vi "PCO_Live.vi"(7 "Message Data":variant, 8 "entrée d'erreur (pas d'erreur)":errorcluster, 9 "Display loop":refnum<queue>, 10 "dup Message Queue":refnum<queue>, 11 "Camera en entrée":refnum<class "Camera.lvclass">) -> (0 "sortie d'erreur":errorcluster, 3 "Camera en sortie":refnum<class "Camera.lvclass">)   [LabVIEW 2026]
uses:
  QMH/Message Queue/Message Cluster.ctl
  <instrlib>/PCO_SDK/File Group 0/vi.lib/Excelitas PCO GmbH/pco.labview/camera/Camera.lvclass
  <instrlib>/PCO_SDK/File Group 0/vi.lib/Excelitas PCO GmbH/pco.labview/camera/Controls/binning.ctl
  Controls/PCO_Config.ctl
  Controls/TypeDef_FGV.ctl
  QMH/Message Queue/Enqueue Message (Single).vi
  QMH/Message Queue/Message Queue.lvlib
panel:
  out "cluster de sortie":T2 {"binning"."mode" items=["sum", "average"]}
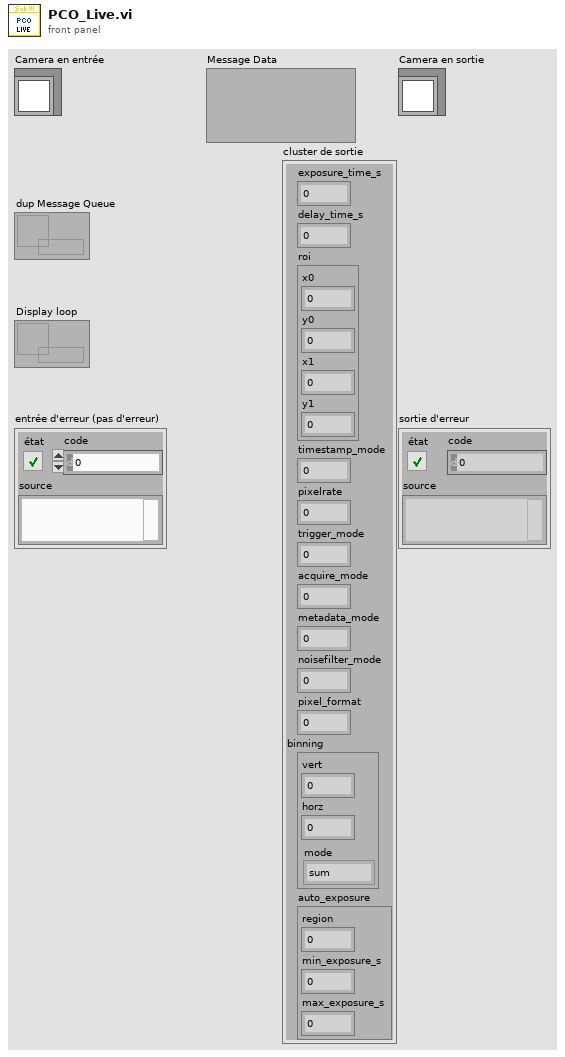
[diagram p1: front panel]
types:
  T1 = typedef "Camera.lvclass/binning.ctl" = cluster{"vert":u16, "horz":u16, "mode":u16}
  T2 = cluster{"exposure_time_s":dbl, "delay_time_s":dbl, "roi":cluster{"x0":u64, "y0":u64, "x1":u64, "y1":u64}, "timestamp_mode":u16, "pixelrate":u32, "trigger_mode":u16, "acquire_mode":u16, "metadata_mode":u16, "noisefilter_mode":u16, "pixel_format":u32, "binning":T1, "auto_exposure":cluster{"region":u16, "min_exposure_s":dbl, "max_exposure_s":dbl}}
  T3 = typedef "PCO_Config.ctl" = cluster{"Exposure time (s)":dbl, "TriggerMode":u16, "ROI X0":u16, "ROI Y0":u16, "ROI X1":u16, "ROI Y1":u16, "Binning":u8}
  T4 = enum16{"sequence", "sequence non blocking", "ring buffer", "fifo", "sequence_dpcore", "sequence_non_blocking_dpcore", "ring_buffer_dpcore", "fifo_dpcore", "tif", "multitif", "pcoraw", "b16", "dicom", "multidicom", "camram_ring", "camram_segment"}
  T5 = typedef "TypeDef_FGV.ctl" = enum16{"Initialize", "Write", "Read"}
  T6 = enum16{"Undefined", "Mono8", "Mono16", "BGRA8", "RGBA8", "BGRA16", "RGBA16", "CompressedMono8"}
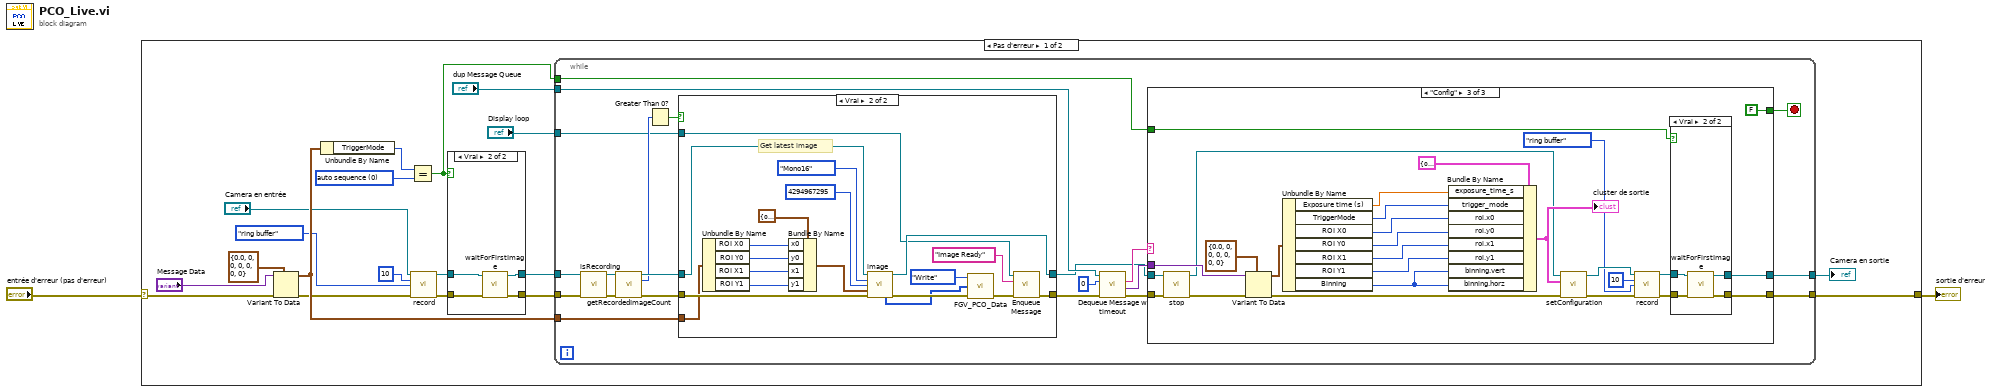
[diagram p0: block diagram]
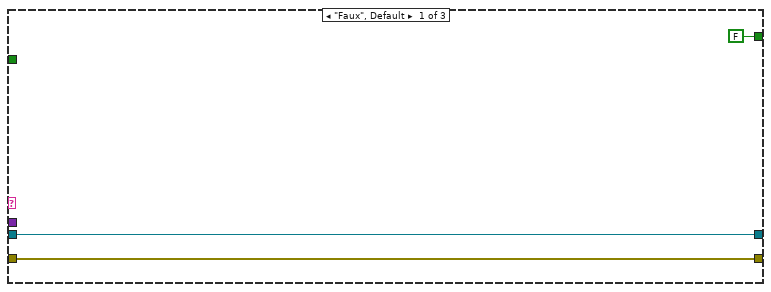
[diagram p2: hidden frame]
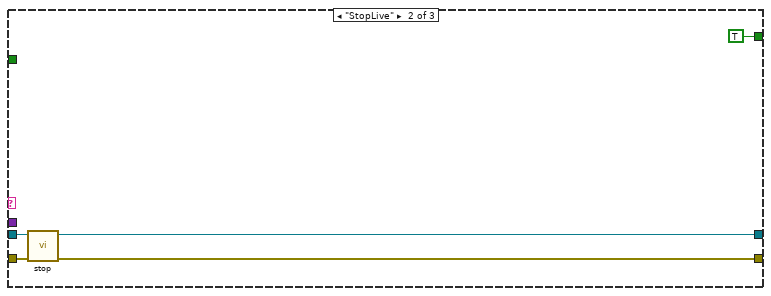
[diagram p3: hidden frame]
diagram:
  n1 = case shown="Pas d'erreur" "entrée d'erreur (pas d'erreur)" {
    selector: "entrée d'erreur (pas d'erreur)" -> [w4 w111]
    tunnel: [w17 w111] -> w2
    frame No Error {
      w10 = u16 0 items=["auto sequence", "software trigger", "external exposure start", "external exposure control"] ("TriggerMode")
      n2 = Variant To Data(error in=w4, type=T3 {"Exposure time (s)"=0.0, "TriggerMode"=0, "ROI X0"=0, "ROI Y0"=0, "ROI X1"=0, "ROI Y1"=0, "Binning"=0} ("PCO_Config"), Variant="Message Data") -> (data=w15:T3, error out=w9:errorcluster)
      n3 = Unbundle By Name(w15) -> ("TriggerMode"=w11:u16)
      n4 = Equal?(x=w11, y=w10) -> (x = y?=w3:bool)
      n5 = call-dynamic "record.vi"("Camera in"="Camera en entrée", "num_images"=u32 10 ("dwImgCount"), "record_mode"=T4."ring buffer", "error in (no error)"=w9) -> ("Camera out"=w20:refnum<class "Camera.lvclass">, "error out"=w19:errorcluster)  [unwired: 10 in]
      n6 = case shown="Vrai" w3 {
        tunnel: w19 -> [w105 w110]
        tunnel: w20 -> [w106 w109]
        tunnel: [w106 w108] -> w14
        tunnel: [w105 w107] -> w13
        frame False {
        }
        frame True {
          n7 = call-dynamic "waitForFirstImage.vi"("error in (no error)"=w110, "Camera in"=w109) -> ("error out"=w107:errorcluster, "Camera out"=w108:refnum<class "Camera.lvclass">)  [unwired: 8 in]
        }
      }
      n8 = while {
        tunnel: w13 -> [w36]
        tunnel: w14 -> [w35]
        tunnel: w15 -> [w34]
        tunnel: "dup Message Queue" -> [w32]
        tunnel: "Display loop" -> [w30]
        tunnel: [w26] -> w17
        tunnel: [w25] -> w18
        tunnel: w3 -> [w22]
        stop <- w24 stop-if-true
        n9 = call-dynamic "isRecording.vi"("Camera in"=w35, "error in (no error)"=w36) -> ("Camera out"=w42:refnum<class "Camera.lvclass">, "error out"=w41:errorcluster)  [unwired: 11 in, 1 out]
        n10 = call-dynamic "getRecordedImageCount.vi"("Camera in"=w42, "error in (no error)"=w41) -> ("Camera out"=w39:refnum<class "Camera.lvclass">, "recorded_image_count"=w37:u32, "error out"=w40:errorcluster)  [unwired: 11 in]
        n11 = Greater Than 0?(x=w37) -> (x > 0?=w38:bool)
        n12 = case shown="Vrai" w38 {
          tunnel: [w84 w90] -> w33
          tunnel: w40 -> [w84 w101]
          tunnel: w39 -> [w85 w100]
          tunnel: [w85 w99] -> w27
          tunnel: w34 -> [_ w98]
          tunnel: w30 -> [_ w92]
          frame False {
          }
          frame True {
            # "Get latest image"
            n13 = Unbundle By Name(w98) -> ("ROI X0"=w97:u16, "ROI Y0"=w96:u16, "ROI X1"=w95:u16, "ROI Y1"=w94:u16)
            n14 = Bundle By Name(cluster=cluster{"x0":u64, "y0":u64, "x1":u64, "y1":u64} {"x0"=0, "y0"=0, "x1"=0, "y1"=0} ("roi"), "x0"=w97, "y0"=w96, "x1"=w95, "y1"=w94) -> (w102:cluster{"x0":u64, "y0":u64, "x1":u64, "y1":u64})
            n15 = call-dynamic "image.vi"("Camera in"=w100, "data_format"=T6."Mono16", "image_index"=u32 4294967295 ("dwImgIdx"), "roi"=w102, "error in (no error)"=w101) -> ("Camera out"=w99:refnum<class "Camera.lvclass">, "raw_image (U16)"=w86:u16[][], "error out"=w88:errorcluster)  [unwired: 2 in, 6 out]
            n16 = call "FGV_PCO_Data.vi"("error in"=w88, "Data"=w86, "Action"=TypeDef_FGV."Write") -> ("error out"=w87:errorcluster)  [unwired: 1 in, 1 out]
            n17 = call-poly "Enqueue Message.vi"("error in (no error)"=w87, "Message"="Image Ready", "Message Queue"=w92) -> ("error out"=w90:errorcluster)  [unwired: 7 in, 1 out]
          }
        }
        n18 = call "Dequeue Message w timeout.vi"("entrée d'erreur (pas d'erreur)"=w33, "timeout en ms (-1)"=0, "Message Queue"=w32) -> ("sortie d'erreur"=w29:errorcluster, "Message Data"=w28:variant, "Message"=w31:string)  [unwired: 5 in, 1 out]
        n19 = case shown="\"Config\"" w31 {
          tunnel: w29 -> [w44 w49 w76]
          tunnel: w28 -> [_ _ w62]
          tunnel: w27 -> [w45 w50 w77]
          tunnel: [w44 w48 w56] -> w26
          tunnel: [w45 w47 w57] -> w25
          tunnel: [FALSE TRUE FALSE] -> w24
          tunnel: w22 -> [_ _ w54]
          frame "Faux", Default {
          }
          frame "StopLive" {
            n20 = call-dynamic "stop.vi"("error in (no error)"=w49, "Camera in"=w50) -> ("error out"=w48:errorcluster, "Camera out"=w47:refnum<class "Camera.lvclass">)  [unwired: 8 in]
          }
          frame "Config" {
            n21 = call-dynamic "stop.vi"("error in (no error)"=w76, "Camera in"=w77) -> ("error out"=w61:errorcluster, "Camera out"=w60:refnum<class "Camera.lvclass">)  [unwired: 8 in]
            n22 = Variant To Data(error in=w61, type=T3 {"Exposure time (s)"=0.0, "TriggerMode"=0, "ROI X0"=0, "ROI Y0"=0, "ROI X1"=0, "ROI Y1"=0, "Binning"=0} ("PCO_Config"), Variant=w62) -> (data=w74:T3, error out=w73:errorcluster)
            n23 = Unbundle By Name(w74) -> ("Exposure time (s)"=w71:dbl, "TriggerMode"=w70:u16, "ROI X0"=w65:u16, "ROI Y0"=w66:u16, "ROI X1"=w67:u16, "ROI Y1"=w68:u16, "Binning"=w69:u8)
            n24 = Bundle By Name(cluster=T2 {"exposure_time_s"=0.1, "delay_time_s"=nan, "roi"={"x0"=18446744073709551615, "y0"=18446744073709551615, "x1"=18446744073709551615, "y1"=18446744073709551615}, "timestamp_mode"=65535, "pixelrate"=4294967295, "trigger_mode"=65535, "acquire_mode"=65535, "metadata_mode"=65535, "noisefilter_mode"=65535, "pixel_format"=4294967295, "binning"={"vert"=65535, "horz"=65535, "mode"=0}, "auto_exposure"={"region"=0, "min_exposure_s"=0.001, "max_exposure_s"=0.1}} ("configuration"), "exposure_time_s"=w71, "trigger_mode"=w70, "roi.x0"=w65, "roi.y0"=w66, "roi.x1"=w67, "roi.y1"=w68, "binning.vert"=w69, "binning.horz"=w69) -> (w72:T2)
            "cluster de sortie" <- w72
            n25 = call-dynamic "setConfiguration.vi"("error in (no error)"=w73, "configuration"=w72, "Camera in"=w60) -> ("error out"=w55:errorcluster, "Camera out"=w59:refnum<class "Camera.lvclass">)  [unwired: 7 in]
            n26 = call-dynamic "record.vi"("Camera in"=w59, "num_images"=u32 10, "record_mode"=T4."ring buffer", "error in (no error)"=w55) -> ("Camera out"=w58:refnum<class "Camera.lvclass">, "error out"=w52:errorcluster)  [unwired: 10 in]
            n27 = case shown="Vrai" w54 {
              tunnel: w58 -> [w79 w83]
              tunnel: [w79 w82] -> w57
              tunnel: [w78 w81] -> w56
              tunnel: w52 -> [w78 w80]
              frame False {
              }
              frame True {
                n28 = call-dynamic "waitForFirstImage.vi"("error in (no error)"=w80, "Camera in"=w83) -> ("error out"=w81:errorcluster, "Camera out"=w82:refnum<class "Camera.lvclass">)  [unwired: 8 in]
              }
            }
          }
        }
      }
      "Camera en sortie" <- w18
    }
    frame Error {
    }
  }
  "sortie d'erreur" <- w2
